vi "Tell Self.vi"(4 "Priority":bool, 10 "Msg":refnum<class "Msg.lvclass">, 11 "Core Actor in":refnum<class "Core Actor.lvclass">) -> (0 "Error out":errorcluster)   [LabVIEW 2025, in "jettl.lvlib" / "Actor.lvlib" / "Core Actor.lvclass"]
uses:
  Core Actor.lvclass
  Msg/Msg.lvclass
  Relation.ctl
  Core Actor.lvclass/Core Actor.ctl
  Attributes/Attributes/Attributes.lvclass
  Actor.lvlib
  Error/Error.lvlib
  Teller/Teller.lvlib
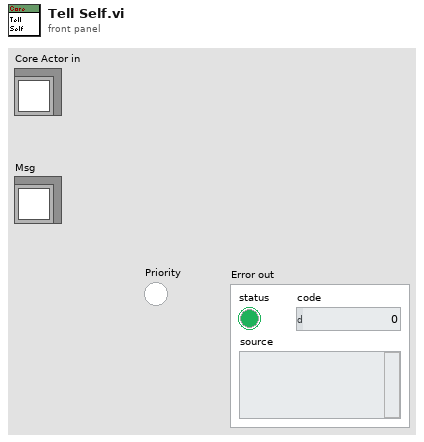
[diagram p1: front panel]
types:
  T1 = typedef "jettl.lvlib/Actor.lvlib/Msg Set.ctl" = set{refnum<class "Msg.lvclass">}
  T2 = typedef "jettl.lvlib/Actor.lvlib/Relation.ctl" = enum16{"Self", "Parent", "Child"}
  T3 = typedef "usereventprio.ctl" = enum32{"high priority", "normal priority"}
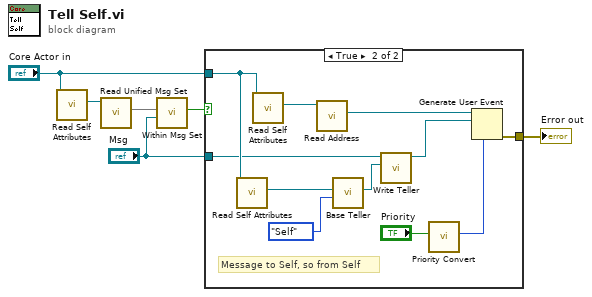
[diagram p0: block diagram]
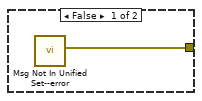
[diagram p2: hidden frame]
diagram:
  n1 = call-dynamic "Read Self Attributes.vi"("Core Actor in"="Core Actor in") -> ("Self Attributes"=w3:refnum<class "Attributes.lvclass">)  [unwired: 10 in]
  n2 = call-dynamic "Read Unified Msg Set.vi"("Attributes in"=w3) -> ("Unified Msg Set"=w2:T1)  [unwired: 10 in]
  n3 = call "Within Msg Set.vi"("Msg"="Msg", "Msg Set"=w2) -> ("Within Msg Set"=w6:bool)  [unwired: 9 in]
  n4 = case shown="True" w6 {
    tunnel: "Core Actor in" -> [_ w18]
    tunnel: "Msg" -> [_ w15]
    tunnel: [w7 w8] -> w1
    frame False {
      n5 = call "Msg Not In Unified Set--error.vi"() -> ("Error"=w7:errorcluster)  [unwired: 11 in]
    }
    frame True {
      # "Message to Self, so from Self"
      n6 = call-dynamic "Read Self Attributes.vi"("Core Actor in"=w18) -> ("Self Attributes"=w14:refnum<class "Attributes.lvclass">)  [unwired: 10 in]
      n7 = call-dynamic "Read Self Attributes.vi"("Core Actor in"=w18) -> ("Self Attributes"=w17:refnum<class "Attributes.lvclass">)  [unwired: 10 in]
      n8 = call-dynamic "Read Address.vi"("Attributes in"=w17) -> ("Address"=w11:refnum<user-event>)  [unwired: 10 in]
      n9 = call "Base Teller.vi"("Relation"=Relation."Self", "Self Attributes"=w14) -> ("Teller"=w16:refnum<class "Teller.lvclass">)  [unwired: 9 in]
      n10 = call-dynamic "Write Teller.vi"("Teller"=w16, "Msg in"=w15) -> ("Msg out"=w10:refnum<class "Msg.lvclass">)  [unwired: 9 in]
      n11 = call "Priority Convert.vi"("Priority"="Priority") -> ("Priority"=w12:T3)  [unwired: 10 in]
      n12 = Generate User Event(priority (normal)=w12, user event=w11, event data cluster=w10) -> (error out=w8:errorcluster)  [unwired: 1 in, 1 out]
    }
  }
  "Error out" <- w1
